vi "find best period - three array.vi"(9 "Array of strobe desired times":dbl[unit][](array[numeric]), 10 "Array of Ch2 desired times":dbl[unit][](array[numeric]), 11 "Array of Ch1 desired times":dbl[unit][](array[numeric])) -> (0 "Array of strobe actual times":dbl[unit][](array[numeric]), 1 "Array of Ch2 \"period-units\"":i32[](array[numeric]), 2 "Array of Ch2 actual times":dbl[unit][](array[numeric]), 3 "Array of Ch1 \"period-units\"":i32[](array[numeric]), 4 "Array of strobe \"period-units\"":i32[](array[numeric]), 5 "Array of Ch1 actual times":dbl[unit][](array[numeric]), 7 "best period":dbl[unit])   [LabVIEW 2015]
doc: "This will find the best period (defined as the one with the minimum squared error), given an array of times from channel 1 and an array of times from channel 2."
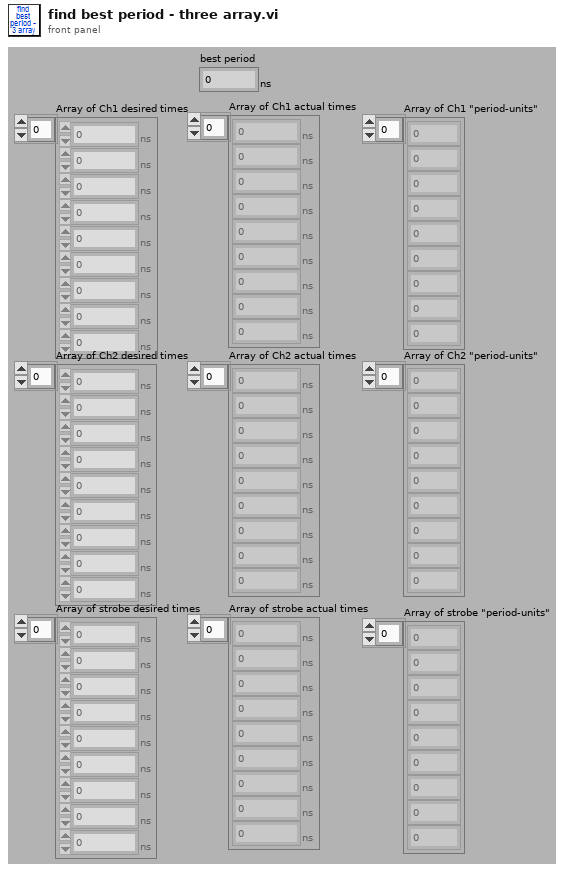
[diagram p1: front panel]
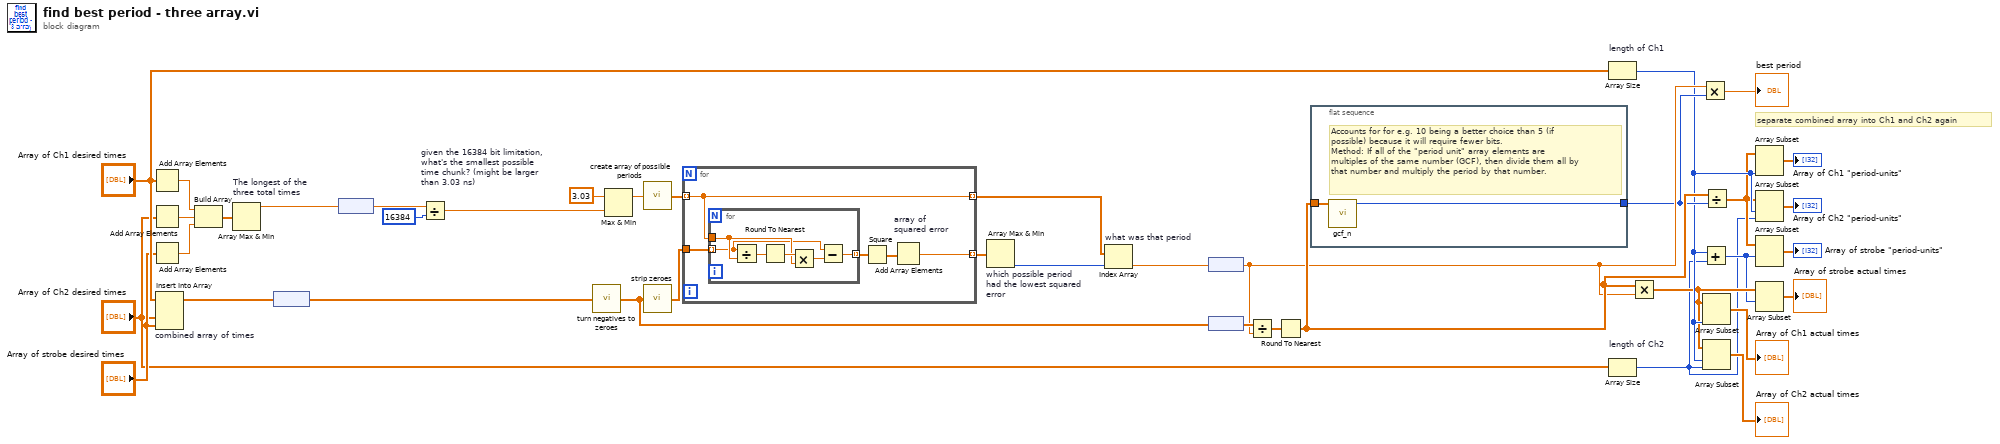
[diagram p0: block diagram]
diagram:
  # "separate combined array into Ch1 and Ch2 again"
  n1 = Add Array Elements(numeric array="Array of Ch1 desired times") -> (sum=w13:dbl[unit])
  n2 = Add Array Elements(numeric array="Array of Ch2 desired times") -> (sum=w12:dbl[unit])
  n3 = Add Array Elements(numeric array="Array of strobe desired times") -> (sum=w11:dbl[unit])
  n4 = Insert Into Array "combined array of times"(array="Array of Ch1 desired times", new element #1="Array of Ch2 desired times", new element #2="Array of strobe desired times") -> (w20:dbl[unit][])  [unwired: 1 in]
  n5 = Build Array(w13, w12, w11) -> (w15:dbl[unit][])
  n6 = Array Max & Min "The longest of the \nthree total times"(array=w15) -> (max value=w10:dbl[unit])  [unwired: 3 out]
  n7 = node(w20) -> (w21:dbl[])
  n8 = node(w10) -> (w34:dbl)
  n9 = Divide "given the 16384 bit limitation, \nwhat's the smallest possible \ntime chunk? (might be larger\nthan 3.03 ns)"(x=w34, y=16384) -> (x/y=w39:dbl)
  n10 = call "turn negatives to zeroes.vi"("Array in"=w21) -> ("Array out"=w27:dbl[])
  n11 = Max & Min(x=3.03, y=w39) -> (max(x,y)=w37:dbl)  [unwired: 1 out]
  n12 = call "create array of possible periods.vi"("starting number"=w37) -> ("array of possible periods"=w38:dbl[])
  n13 = call "strip zeroes.vi"("Array in"=w27) -> ("Array out"=w28:dbl[])
  n14 = for {
    tunnel: w28 -> [w44]
    tunnel: [w41] -> w32 mode=indexing
    tunnel: [w43] -> w30 mode=indexing
    tunnel: w38 -> [w43] mode=indexing
    n15 = for {
      tunnel: w44 -> [w47] mode=indexing
      tunnel: w43 -> [w48]
      tunnel: [w45] -> w40 mode=indexing
      n16 = Divide(x=w47, y=w48) -> (x/y=w50:dbl)
      n17 = Round To Nearest(number=w50) -> (nearest integer value=w49:dbl)
      n18 = Multiply(x=w49, y=w48) -> (x*y=w46:dbl)
      n19 = Subtract(x=w47, y=w46) -> (x-y=w45:dbl)
    }
    n20 = Square(x=w40) -> (x^2=w42:dbl[])
    n21 = Add Array Elements "array of \nsquared error"(numeric array=w42) -> (sum=w41:dbl)
  }
  n22 = Array Max & Min "which possible period\nhad the lowest squared \nerror"(array=w32) -> (min index (indices)=w31:i32)  [unwired: 3 out]
  n23 = Index Array "what was that period"(array=w30, index=w31) -> (element=w33:dbl)
  n24 = node(w33) -> (w24:dbl[unit])
  n25 = node(w27) -> (w26:dbl[unit][])
  n26 = Divide(x=w26, y=w24) -> (x/y=w29:dbl[])
  n27 = Round To Nearest(number=w29) -> (nearest integer value=w25:dbl[])
  n28 = flat-sequence {
    tunnel: w25 -> [w52]
    tunnel: [w51] -> w23
    frame #0 {
      # "Accounts for for e.g. 10 being a better choice than 5 (if\npossible) because it will require fewer bits. \nMethod: If all of the \"period unit\" array elements are\nmultiples of the same number (GCF), then divide them all by\nthat number and multiply the period by that number."
      n29 = call "gcf_n.vi"("Values"=w52) -> ("GCF"=w51:i32)  [unwired: 1 in, 9 out]
    }
  }
  n30 = Array Size "length of Ch1"(array="Array of Ch1 desired times") -> (size(s)=w7:i32)
  n31 = Array Size "length of Ch2"(array="Array of Ch2 desired times") -> (size(s)=w1:i32)
  n32 = Multiply(x=w25, y=w24) -> (x*y=w6:dbl[unit][])
  n33 = Multiply(x=w24, y=w23) -> (x*y=→"best period":dbl[unit])
  n34 = Add(x=w7, y=w1) -> (x+y=w3:i32)
  n35 = Divide(x=w25, y=w23) -> (x/y=w4:dbl[])
  n36 = Array Subset(array=w6, length=w7) -> (→"Array of Ch1 actual times":dbl[unit][])  [unwired: 1 in]
  n37 = Array Subset(array=w6, index=w7, length=w1) -> (→"Array of Ch2 actual times":dbl[unit][])
  n38 = Array Subset(array=w4, length=w7) -> (→"Array of Ch1 \"period-units\"":dbl[])  [unwired: 1 in]
  n39 = Array Subset(array=w4, index=w7, length=w1) -> (→"Array of Ch2 \"period-units\"":dbl[])
  n40 = Array Subset(array=w4, index=w3) -> (→"Array of strobe \"period-units\"":dbl[])  [unwired: 1 in]
  n41 = Array Subset(array=w6, index=w3) -> (→"Array of strobe actual times":dbl[unit][])  [unwired: 1 in]
